vi "LEO PROVA MINCHIATA.vi"() -> ()   [LabVIEW 2014]
uses:
  <vilib>/Platform/TimedLoop/XDataNode/timing_clust.ctl
  <vilib>/Platform/TimedLoop/XDataNode/nitl_modes.ctl
  <vilib>/Platform/TimedLoop/XDataNode/wakeup.ctl
  <vilib>/rvi/Analysis/measure/FFT/simModelSupport/niFPGA FFT Streaming Sim Properties.ctl
  <vilib>/rvi/Analysis/measure/FFT/simModelSupport/niFPGA FFT Sim Stream Group Properties.ctl
  <vilib>/rvi/Analysis/measure/FFT/simModelSupport/niFPGA FFT Sim Types.ctl
  <vilib>/rvi/Analysis/measure/FFT/simModelSupport/niFpgaFFTSimArithmeticProperties.ctl
  <vilib>/rvi/Analysis/measure/FFT/simModelSupport/niFpgaFFTSimDfxp.ctl
  <vilib>/fxp/LVFixedPointQuantizationPolicyTypeDef.ctl
  <vilib>/rvi/Analysis/measure/FFT/XNode/niFpgaFFTButterflyDelays.ctl
  <vilib>/rvi/Emulation/niFpgaSctlEmulationGetInTimedLoop.vi
  <vilib>/rvi/Emulation/niFpgaEmulationReportErrorSimple.vi
  <vilib>/rvi/Emulation/niFpgaGetClockAttributes.vi
  <vilib>/rvi/Emulation/niFpgaCriticalErrorInLSC.vi
  <vilib>/rvi/Emulation/niFpgaEmulationIsFPGAContextNoSignature.vi
  <vilib>/rvi/errors/niFpgaSetErrorForExecOnDevCompSimple.vi
  <vilib>/rvi/eio/common/nirviEmuReportErrorAndStop.vi
  <vilib>/rvi/DataTransferAndStorage/Container/Common/niFpgaContainerGetUniqueNameForEmu.vi
  <vilib>/rvi/FIFO/Fifo_Resource/nirvififoEmulationSetSize.vi
  <vilib>/rvi/FIFO/Fifo_Resource/nirviFifoEmulationQueueMgr.vi
  <instcachedir>/0/nirviFifoEmulationQueueMgr_E5CAEC123FF24DC58D834DCA3CDAA9B5.lvgen/nirviFifoEmulationQueueMgr_E5CAEC123FF24DC58D834DCA3CDAA9B5_012.vi
  <vilib>/rvi/FIFO/Fifo_Resource/nirvififoEmulationCreateLock.vi
  <vilib>/rvi/Emulation/niFpgaProcessEmulError.vi
  <vilib>/rvi/FIFO/Fifo_Resource/nirvififoEmulationObtainLock.vi
  <vilib>/rvi/FIFO/Fifo_Resource/nirvififoEmulationReleaseLock.vi
  <vilib>/rvi/occurrence/nirviWaitOnOccurrenceBase.vi
  <vilib>/rvi/errors/nirviReportUnexpectedCaseInternalError.vi
  <vilib>/rvi/errors/nirviReportUnexpectedCaseInternalError (U32).vi
  <vilib>/rvi/Memory/Memory_Emulation/niFpgaMemoryEmulationCacheClearOnFirstRun.vi
  <vilib>/rvi/Memory/Memory_Emulation/nirvimemoryEmulationManagerCache_MakeExclusive.vi
  <vilib>/rvi/Memory/Memory_Emulation/niFpgaMemoryEmulationValidateCache.vi
  <vilib>/rvi/Memory/Memory_Emulation/nirvimemoryEmulationManagerCache_InsertValue.vi
  <vilib>/Utility/error.llb/Clear Errors.vi
  <vilib>/rvi/Memory/Memory_Emulation/nirvimemoryEmulationManagerCache_ReleaseExclusive.vi
  <vilib>/rvi/Memory/Memory_Emulation/nirvimemoryEmulationManagerCache_GetValue.vi
  <vilib>/rvi/Memory/Memory_Emulation/nirvimemoryEmulationManagerCache_SetValue.vi
  <instcachedir>/0/nirviFifoEmulationQueueMgr_E5CAEC123FF24DC58D834DCA3CDAA9B5.lvgen/nirviFifoEmulationQueueMgr_E5CAEC123FF24DC58D834DCA3CDAA9B5_010.vi
  <vilib>/rvi/FIFO/Fifo_Resource/nirvififoEmulationDetermineInputValidOut.vi
  <vilib>/rvi/Memory/Memory_Emulation/nirvimemoryFastEmulation.vi
  <vilib>/rvi/Memory/Memory_Emulation/nirvimemoryEmulation.vi
  <vilib>/rvi/Analysis/measure/FFT/simModelSupport/niFpgaFFTSimModelStreamingCore.vi
  <vilib>/rvi/interface/RandomDataEmulation/niFpgaRandomDataHandleErrors.vi
  <vilib>/rvi/eio/common/nirviEmuTemplateMethod_errors.vi
  <vilib>/Platform/TimedLoop/XDataNode/XDataNode.xnode
  <vilib>/rvi/DataTransferAndStorage/Container/XNode/niFpgaContainer.xnode
  <vilib>/rvi/FIFO/Fifo_Resource/nirvififoEmulationRead.vi
  <vilib>/rvi/DataTransferAndStorage/Register/Emulation/niFpgaRegisterEmulation.vi
  <vilib>/rvi/FIFO/Fifo_Resource/nirvififoEmulationWrite.vi
  <vilib>/rvi/FIFO/Fifo_Resource/nirvififoEmulationGetNumberOfElementsToWrite.vi
  <vilib>/rvi/Analysis/measure/FFT/XNode/niFpgaFFT.xnode
  <vilib>/rvi/interface/RandomDataEmulation/nirviRandomDataFpgaReadWriteTemplate.vi
  <vilib>/eio/EIOMethodNode/EIOMethodNode.xnode
  <vilib>/Platform/TimedLoop/XDataNode/XDNodeRunTimeDep.lvlib
panel:
  in  "snapshot":bool
  in  "first bin":i32=4
  in  "last bin":i32=251
  in  "lower limit 2":u32=682
  in  "lower limit 1":u32=57
  in  "upper limit 2":u32=1194
  in  "upper limit 1":u32=569
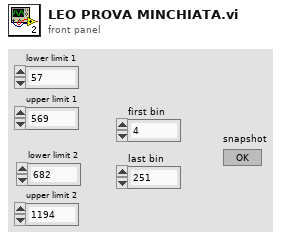
[diagram p1: front panel]
types:
  T1 = typedef "XDNodeRunTimeDep.lvlib/timing_clust.ctl" = cluster{"Expected End [f-1]":u64, "Actual End [f-1]":u64, "Finished Late? [f-1]":bool, "Expected End [i-1]":u64, "Actual End [i-1]":u64, "Finished Late? [i-1]":bool, "Expected Start [i]":u64, "Actual Start [i]":u64, "Expected Start [f]":u64, "Actual Start [f]":u64, "Source Name":string, "Structure Name":string, "Period":i64, "Deadline":i64, "Offset":i64, "Start":i64, "Priority":i32, "Timeout":i32, "Mode":T2, "Wakeup Reason":T3, "Error":errorcluster, "Source Type":string, "Secondary Source Type":string, "Global End Time":u64, "Global Start Time":u64, "Frame Duration":u64, "Iteration Duration":u64, "Assigned CPU":i32, "I/O Scan Engine Mode":u32}
  T2 = typedef "XDNodeRunTimeDep.lvlib/nitl_modes.ctl" = enum32{"No Change", "Process missed periods, maintain original phase", "Discard missed periods, maintain original phase", "Process missed periods, ignore original phase", "Discard missed periods, ignore original phase"}
  T3 = typedef "XDNodeRunTimeDep.lvlib/wakeup.ctl" = enum32{"Normal", "Aborted", "Asynchronous wakeup", "Timing source error", "Timed loop error", "Timeout"}
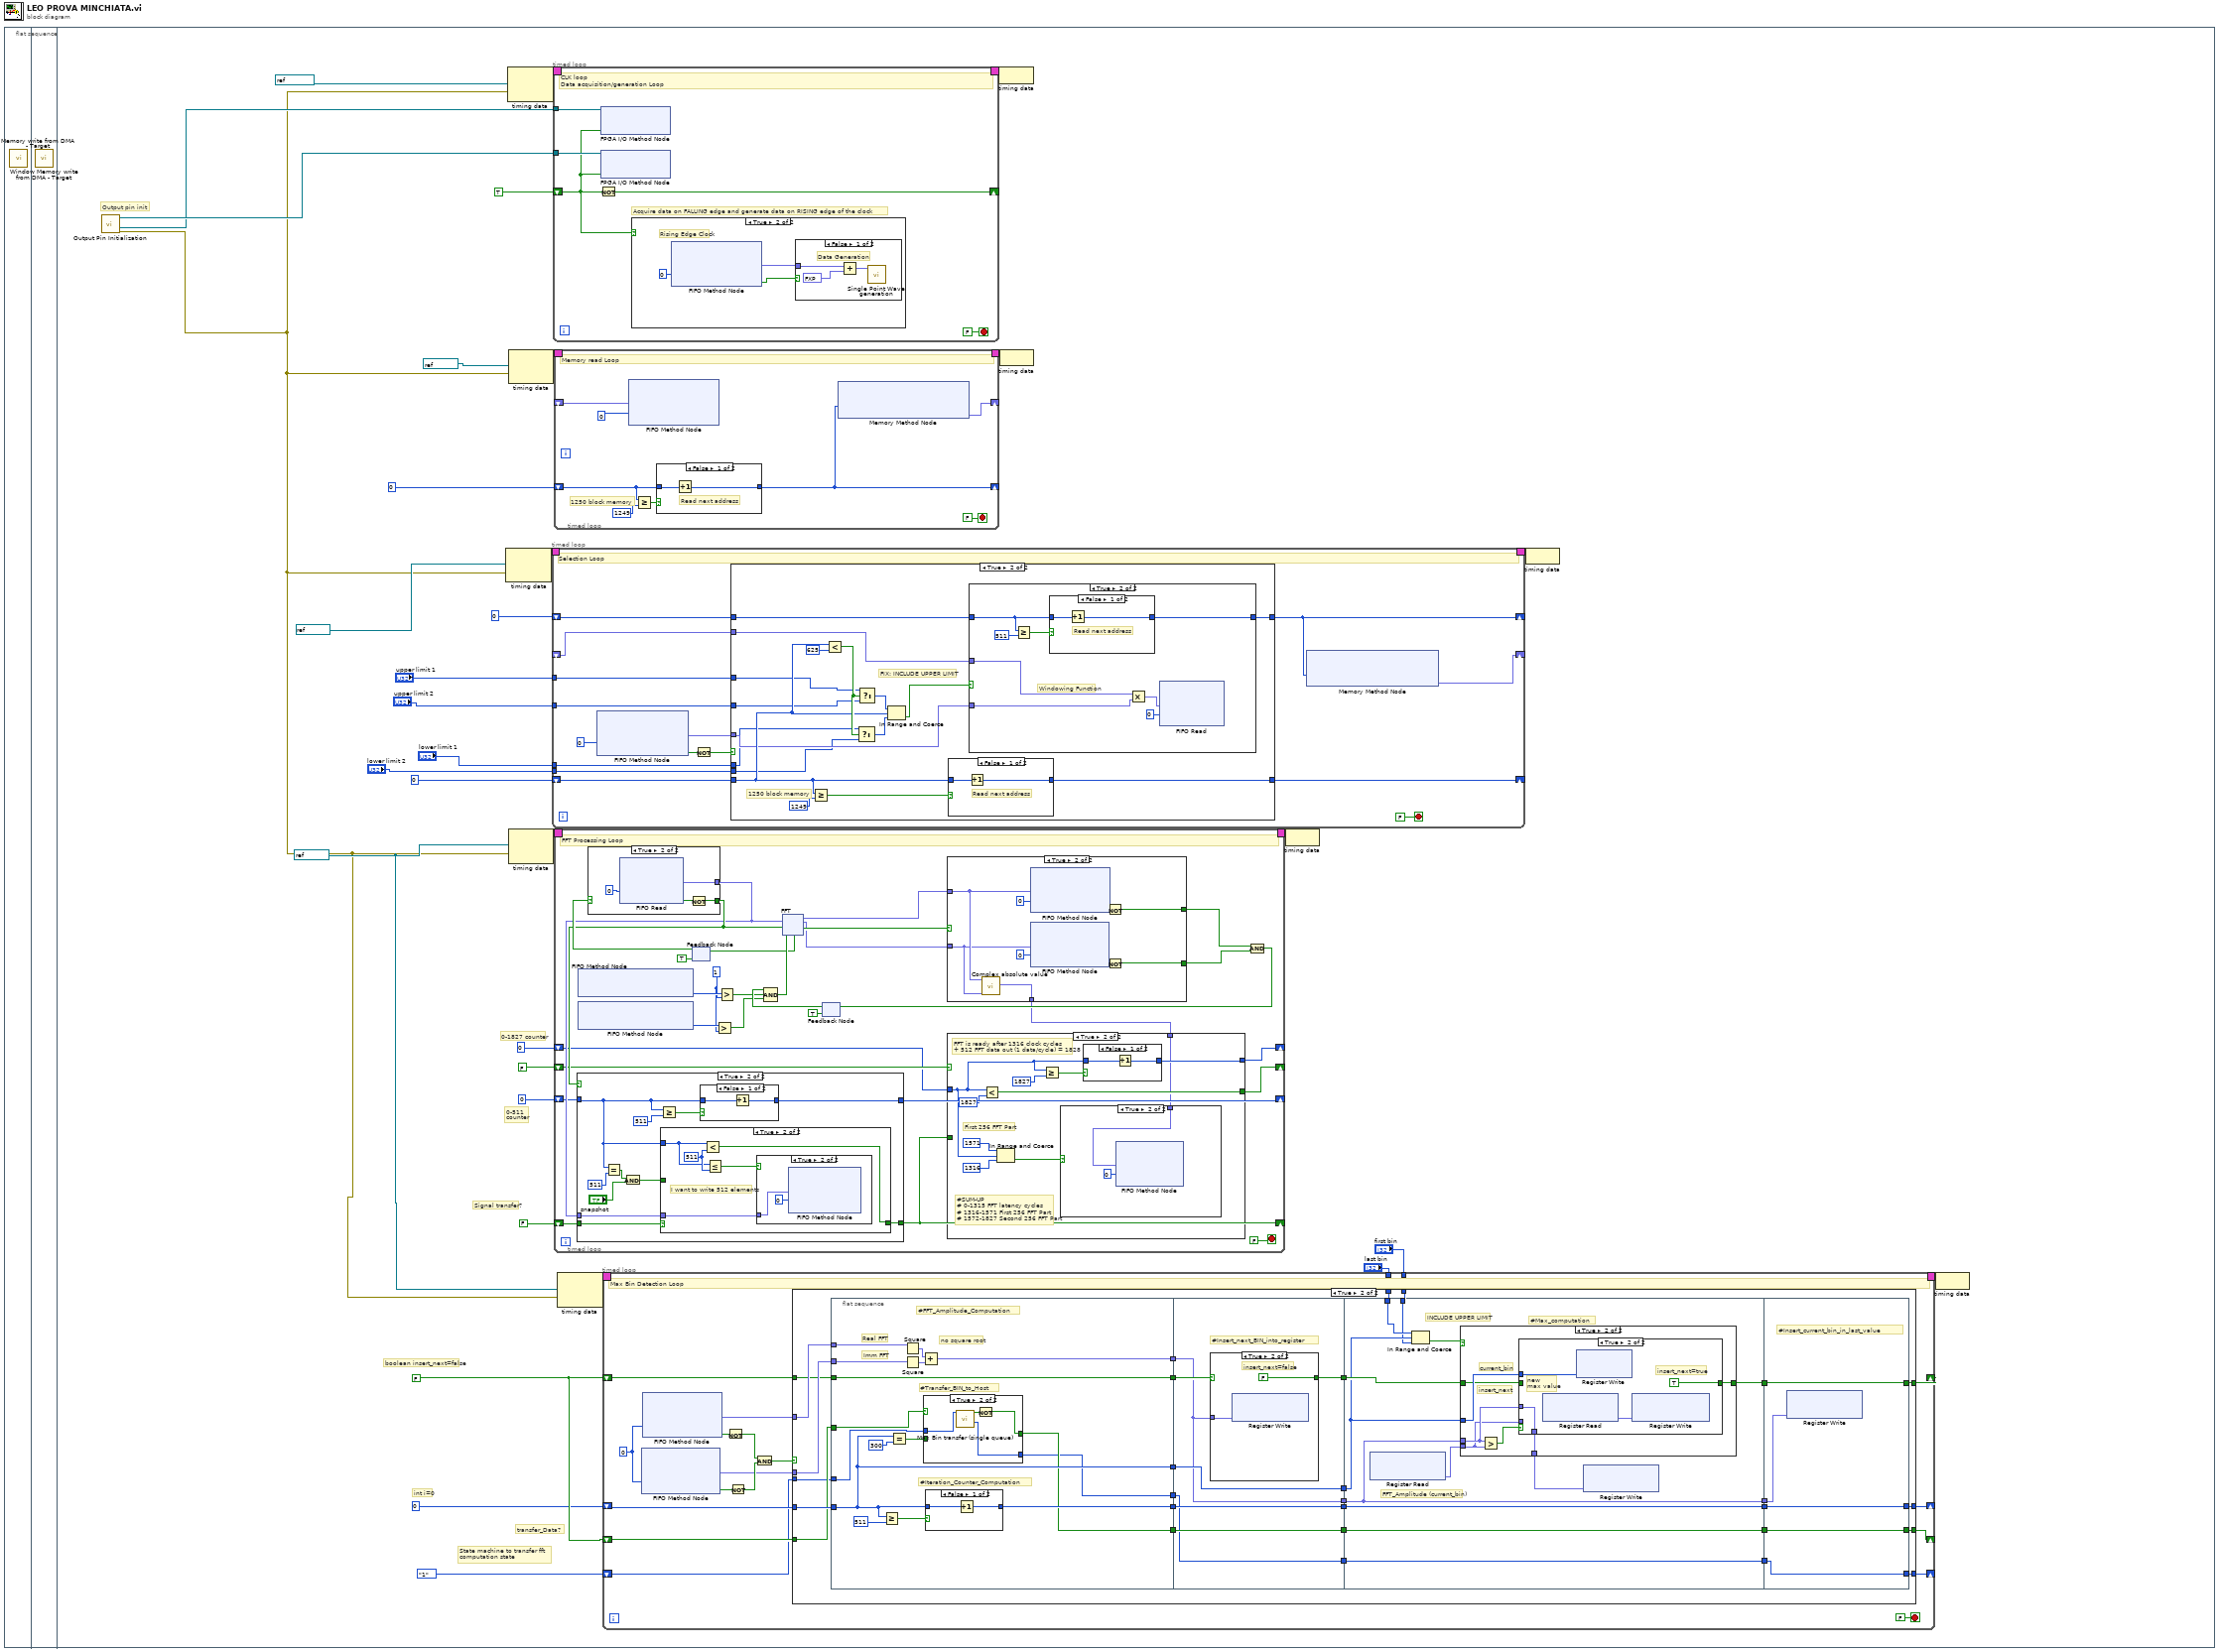
[diagram p0: block diagram]
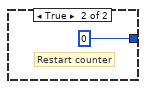
[diagram p4: hidden frame]
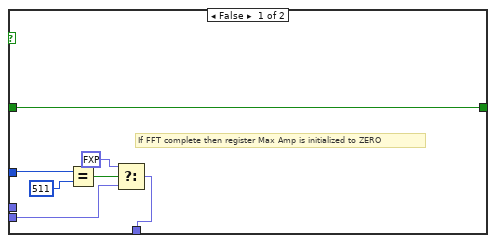
[diagram p6: hidden frame]
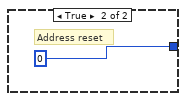
[diagram p10: hidden frame]
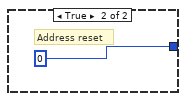
[diagram p11: hidden frame]
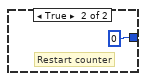
[diagram p14: hidden frame]
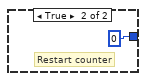
[diagram p18: hidden frame]
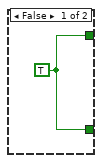
[diagram p19: hidden frame]
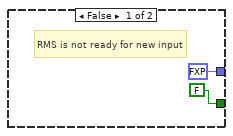
[diagram p20: hidden frame]
diagram:
  n1 = flat-sequence {
    frame #0 {
      n2 = call "Memory write from DMA - Target.vi"() -> ()  [unwired: 12 in]
    }
    frame #1 {
      n3 = call "Window Memory write from DMA - Target.vi"() -> ()  [unwired: 12 in]
    }
    frame #2 {
      w7 = FALSE
      w16 = refnum<k21> "50MHz" ("Source Name")
      # "0-1827 counter"
      # "0-511\ncounter"
      # "Signal transfer?"
      # "State machine to transfer fft\ncomputation state"
      # "transfer_Data?"
      # "int i=0"
      # "boolean insert_next=false"
      # "Output pin init"
      n4 = call "Output Pin Initialization.vi"() -> ("error out"=w15:errorcluster, "I/O Out Clock DAC (pin16)"=w19:refnum<k21>, "I/O Out Clock ADC (pin17)"=w20:refnum<k21>)  [unwired: 8 in]
      n5 = node-c288(refnum<k21> "50MHz" ("Source Name"), w15) -> (w28:T1)
      n6 = node-c288(refnum<k21> "100MHz" ("Source Name"), w15) -> (w34:T1)
      n7 = node-c288(refnum<k21> "50MHz" ("Source Name"), w15) -> (w32:T1)
      n8 = node-c288(w16, w15) -> (w30:T1)
      n9 = timed-loop {
        timing: w28 -> [_]
        timing-out: [_] -> w27
        shift-right: [w179] -> _
        shift-left: u32 0 -> [w178]
        tunnel: "upper limit 1" -> [w173]
        tunnel: "upper limit 2" -> [w172]
        tunnel: "lower limit 1" -> [w171]
        tunnel: "lower limit 2" -> [w170]
        shift-right: [w166] -> _
        shift-left: u32 0 -> [w169]
        shift-right: [w167] -> _
        shift-left: _ -> [w168]
        stop <- FALSE stop-if-true
        # "Selection Loop"
        n10 = xnode ("FIFO Method Node")("Timeout"=0) -> ("Element"=w175:fxp<+/-,12,12>, "Timed Out?"=w176:bool)  [unwired: 1 in, 1 out]
        n11 = Not(x=w176) -> (.not. x?=w177:bool)
        n12 = case shown="True" w177 {
          tunnel: [w182 w197] -> w179
          tunnel: w178 -> [w182 w192]
          tunnel: w175 -> [_ w190]
          tunnel: w173 -> [_ w189]
          tunnel: w172 -> [_ w188]
          tunnel: w171 -> [_ w187]
          tunnel: w170 -> [_ w186]
          tunnel: w169 -> [w181 w183]
          tunnel: [w181 w185] -> w166
          tunnel: w168 -> [_ w184]
          frame False {
          }
          frame True {
            # "FIX: INCLUDE UPPER LIMIT"
            # "1250 block memory"
            n13 = Greater Or Equal?(x=w192, y=u32 1249) -> (x >= y?=w198:bool)
            n14 = Less?(x=w192, y=u32 625) -> (x < y?=w193:bool)
            n15 = Select(t=w187, s=w193, f=w186) -> (s? t:f=w195:u32)
            n16 = Select(t=w189, s=w193, f=w188) -> (s? t:f=w196:u32)
            n17 = In Range and Coerce(upper limit=w196, x=w192, lower limit=w195) -> (In Range?=w191:bool)  [unwired: 1 out]
            n18 = case shown="False" w198 {
              tunnel: w192 -> [w213 _]
              tunnel: [w212 u32 0] -> w197
              frame False {
                # "Read next address"
                n19 = Increment(x=w213) -> (x+1=w212:u32)
              }
              frame True {
                # "Address reset"
              }
            }
            n20 = case shown="True" w191 {
              tunnel: w190 -> [_ w201]
              tunnel: w183 -> [w200 w206]
              tunnel: [w200 w208] -> w185
              tunnel: w184 -> [_ w204]
              frame False {
              }
              frame True {
                # "Windowing Function"
                n21 = Greater Or Equal?(x=w206, y=u32 511) -> (x >= y?=w207:bool)
                n22 = case shown="False" w207 {
                  tunnel: w206 -> [w210 _]
                  tunnel: [w209 u32 0] -> w208
                  frame False {
                    # "Read next address"
                    n23 = Increment(x=w210) -> (x+1=w209:u32)
                  }
                  frame True {
                    # "Address reset"
                  }
                }
                n24 = Multiply(x=w204, y=w201) -> (x*y=w202:fxp<+/-,12,12>)
                n25 = xnode ("FIFO Read")("Element"=w202, "Timeout"=0) -> ()  [unwired: 1 in, 2 out]
              }
            }
          }
        }
        n26 = xnode ("Memory Method Node")("Address"=w166) -> ("Data"=w167:fxp<+,8,1>)  [unwired: 1 in, 1 out]
      }
      n27 = timed-loop {
        timing: w34 -> [_]
        timing-out: [_] -> w33
        shift-right: [w361] -> _
        shift-left: TRUE -> [w359]
        tunnel: w19 -> [w363]
        tunnel: w20 -> [w360]
        stop <- FALSE stop-if-true
        # "Acquire data on FALLING edge and generate data on RISING edge of the clock"
        # "CLK loop\nData acquisition/generation Loop"
        n28 = Not(x=w359) -> (.not. x?=w361:bool)
        n29 = xnode "FPGA I/O Method Node"("FPGA I/O In"=w363, "Data"=w359) -> ()  [unwired: 1 out]
        n30 = xnode "FPGA I/O Method Node"("FPGA I/O In"=w360, "Data"=w359) -> ()  [unwired: 1 out]
        n31 = case shown="True" w359 {
          frame False {
            # "Falling Edge Clock"
            n32 = call "Single Acquisition.vi"() -> ("Out"=w365:fxp<+/-,12,12>)  [unwired: 10 in, 1 out]
            n33 = xnode ("FIFO Method Node")("Element"=w365, "Timeout"=0) -> ()  [unwired: 1 in, 2 out]
          }
          frame True {
            # "Rising Edge Clock"
            n34 = xnode ("FIFO Method Node")("Timeout"=0) -> ("Element"=w366:fxp<+/-,12,12>, "Timed Out?"=w367:bool)  [unwired: 1 in, 1 out]
            n35 = case shown="False" w367 {
              tunnel: w366 -> [w371 _]
              frame False {
                # "Data Generation"
                n36 = Add(x=w371, y=fxp<+,12,12> 2048.0) -> (x+y=w369:fxp<+/-,14,14>)
                n37 = call "Single Point Wave generation.vi"("Data To Write"=w369) -> ()  [unwired: 10 in, 1 out]
              }
              frame True {
                # "FPGA memory slow"
              }
            }
          }
        }
      }
      n38 = timed-loop {
        timing: w32 -> [_]
        timing-out: [_] -> w31
        shift-right: [w341] -> _
        shift-left: u32 0 -> [w345]
        shift-right: [w343] -> _
        shift-left: _ -> [w342]
        stop <- FALSE stop-if-true
        # "1250 block memory"
        # "Memory read Loop"
        n39 = xnode ("FIFO Method Node")("Element"=w342, "Timeout"=0) -> ()  [unwired: 1 in, 2 out]
        n40 = Greater Or Equal?(x=w345, y=u32 1249) -> (x >= y?=w347:bool)
        n41 = case shown="False" w347 {
          tunnel: w345 -> [w350 _]
          tunnel: [w349 u32 0] -> w341
          frame False {
            # "Read next address"
            n42 = Increment(x=w350) -> (x+1=w349:u32)
          }
          frame True {
            # "Address reset"
          }
        }
        n43 = xnode ("Memory Method Node")("Address"=w341) -> ("Data"=w343:fxp<+/-,12,12>)  [unwired: 1 in, 1 out]
      }
      n44 = timed-loop {
        timing: w30 -> [_]
        timing-out: [_] -> w29
        shift-right: [w227] -> _
        shift-left: FALSE -> [w230]
        shift-right: [w231] -> _
        shift-left: i16 0 -> [w228]
        shift-right: [w226] -> _
        shift-left: FALSE -> [w225]
        shift-right: [w223] -> _
        shift-left: i16 0 -> [w224]
        stop <- FALSE stop-if-true
        w235 = u32 1 ("y")
        # "FFT Processing Loop"
        n45 = xnode ("FIFO Method Node")() -> ("Number of Elements to Write"=w237:u32)  [unwired: 1 in, 1 out]
        n46 = xnode ("FIFO Method Node")() -> ("Number of Elements to Write"=w236:u32)  [unwired: 1 in, 1 out]
        n47 = feedback #1(TRUE ("ready for input")) -> (w250:bool)
        n48 = case shown="True" w250 {
          tunnel: [FALSE w333] -> w232
          tunnel: [fxp<+/-,12,12> 0.0 ("Element") w330] -> w229
          frame False {
            # "RMS is not ready for new input"
          }
          frame True {
            n49 = xnode ("FIFO Read")("Timeout"=0) -> ("Element"=w330:fxp<+/-,12,12>, "Timed Out?"=w332:bool)  [unwired: 1 in, 1 out]
            n50 = Not(x=w332) -> (.not. x?=w333:bool)
          }
        }
        n51 = case shown="True" w232 {
          tunnel: w228 -> [w269 w273]
          tunnel: [w269 w278] -> w231
          tunnel: w230 -> [w268 w271]
          tunnel: [w268 w272] -> w227
          tunnel: w229 -> [_ w270]
          frame False {
          }
          frame True {
            n52 = Equal?(x=w273, y=i16 511) -> (x = y?=w277:bool)
            n53 = And(x=w277, y="snapshot") -> (x .and. y?=w274:bool)
            n54 = Greater Or Equal?(x=w273, y=i16 511) -> (x >= y?=w279:bool)
            n55 = case shown="True" w271 {
              tunnel: w274 -> [w281 _]
              tunnel: w273 -> [_ w282]
              tunnel: [w281 w286] -> w272
              tunnel: w270 -> [_ w284]
              frame False {
              }
              frame True {
                w283 = i16 511 ("y")
                # "I want to write 512 elements"
                n56 = Less?(x=w282, y=w283) -> (x < y?=w286:bool)
                n57 = Less Or Equal?(x=w282, y=w283) -> (x <= y?=w285:bool)
                n58 = case shown="True" w285 {
                  tunnel: w284 -> [_ w287]
                  frame False {
                  }
                  frame True {
                    n59 = xnode ("FIFO Method Node")("Element"=w287, "Timeout"=0) -> ()  [unwired: 1 in, 2 out]
                  }
                }
              }
            }
            n60 = case shown="False" w279 {
              tunnel: w273 -> [w290 _]
              tunnel: [w289 i16 0] -> w278
              frame False {
                n61 = Increment(x=w290) -> (x+1=w289:i16)
              }
              frame True {
                # "Restart counter"
              }
            }
          }
        }
        n62 = Greater?(x=w236, y=w235) -> (0:w233:bool)
        n63 = Greater?(x=w237, y=w235) -> (0:w234:bool)
        n64 = feedback #2(TRUE) -> (w246:bool)
        n65 = Compound Arithmetic op=AND(w246, w234, w233) -> (w245:bool)
        n66 = xnode "FFT"("real data in"=w229, "input valid"=w232, "ready for output"=w245) -> ("ready for input"=w244:bool, "real data out"=w242:fxp<+/-,22,22>, "imaginary data out"=w241:fxp<+/-,22,22>, "output valid"=w243:bool)  [unwired: 2 in, 1 out]
        n67 = feedback-in #1(w244) -> ()
        n68 = case shown="True" w243 {
          tunnel: w242 -> [_ w321]
          tunnel: w241 -> [_ w320]
          tunnel: [w318 w327] -> w240
          tunnel: [w318 w326] -> w239
          tunnel: [_ w319] -> w222
          frame False {
            w318 = TRUE
          }
          frame True {
            n69 = call "Complex absolute value.vi"("Im"=w320, "Re"=w321) -> ("Square Absolute Value"=w319:fxp<+,44,44>)  [unwired: 9 in]
            n70 = xnode ("FIFO Method Node")("Element"=w321, "Timeout"=0) -> ("Timed Out?"=w322:bool)  [unwired: 1 in, 1 out]
            n71 = xnode ("FIFO Method Node")("Element"=w320, "Timeout"=0) -> ("Timed Out?"=w323:bool)  [unwired: 1 in, 1 out]
            n72 = Not(x=w322) -> (.not. x?=w327:bool)
            n73 = Not(x=w323) -> (.not. x?=w326:bool)
          }
        }
        n74 = case shown="True" w225 {
          tunnel: w227 -> [w252 _]
          tunnel: [w252 w262] -> w226
          tunnel: w224 -> [w251 w255]
          tunnel: [w251 w258] -> w223
          tunnel: w222 -> [_ w253]
          frame False {
          }
          frame True {
            # "First 256 FFT Part"
            # "#SUM-UP\n# 0-1315 FFT latency cycles\n# 1316-1571 First 256 FFT Part\n# 1572-1827 Second 256 FFT Part"
            # "FFT is ready after 1316 clock cycles\n+ 512 FFT data out (1 data/cycle) = 1828"
            n75 = Less?(x=w255, y=i16 1827) -> (x < y?=w262:bool)
            n76 = In Range and Coerce(upper limit=i16 1571, x=w255, lower limit=i16 1316 ("y")) -> (In Range?=w254:bool)  [unwired: 1 out]
            n77 = Greater Or Equal?(x=w255, y=i16 1827) -> (x >= y?=w259:bool)
            n78 = case shown="True" w254 {
              tunnel: w253 -> [_ w264]
              frame False {
              }
              frame True {
                n79 = xnode ("FIFO Method Node")("Element"=w264, "Timeout"=0) -> ()  [unwired: 1 in, 2 out]
              }
            }
            n80 = case shown="False" w259 {
              tunnel: w255 -> [w266 _]
              tunnel: [w265 i16 0] -> w258
              frame False {
                n81 = Increment(x=w266) -> (x+1=w265:i16)
              }
              frame True {
                # "Restart counter"
              }
            }
          }
        }
        n82 = Compound Arithmetic op=AND(w240, w239) -> (w238:bool)
        n83 = feedback-in #2(w238) -> ()
      }
      n84 = node-c288(w16, w15) -> (w26:T1)
      n85 = timed-loop {
        shift-right: [w45] -> _
        shift-left: 0 ("Timeout") -> [w46]
        shift-right: [w43] -> _
        shift-left: w7 -> [w44]
        timing: w26 -> [_]
        timing-out: [_] -> w25
        tunnel: "last bin" -> [w41]
        tunnel: "first bin" -> [w40]
        shift-right: [w37] -> _
        shift-left: w7 -> [w38]
        shift-right: [w35] -> _
        shift-left: enum16{"1", "2", "3", "4"}."1" ("Enum") -> [w36]
        stop <- FALSE stop-if-true
        w39 = 0 ("Timeout")
        # "Max Bin Detection Loop"
        n86 = xnode ("FIFO Method Node")("Timeout"=w39) -> ("Element"=w47:fxp<+/-,22,22>, "Timed Out?"=w52:bool)  [unwired: 1 in, 1 out]
        n87 = xnode ("FIFO Method Node")("Timeout"=w39) -> ("Element"=w48:fxp<+/-,22,22>, "Timed Out?"=w53:bool)  [unwired: 1 in, 1 out]
        n88 = Not(x=w53) -> (.not. x?=w51:bool)
        n89 = Not(x=w52) -> (.not. x?=w50:bool)
        n90 = And(x=w51, y=w50) -> (x .and. y?=w49:bool)
        n91 = case shown="True" w49 {
          tunnel: w48 -> [_ w86]
          tunnel: w47 -> [_ w85]
          tunnel: w46 -> [w57 w83]
          tunnel: [w57 w70] -> w45
          tunnel: w44 -> [w56 w77]
          tunnel: [w56 w72] -> w43
          tunnel: w41 -> [_ w69]
          tunnel: w40 -> [_ w68]
          tunnel: w38 -> [w55 w67]
          tunnel: [w55 w66] -> w37
          tunnel: w36 -> [w54 w62]
          tunnel: [w54 w58] -> w35
          frame False {
            # "Data are NOT ready in Target Real FFT and Target Imm FFT FIFOs"
          }
          frame True {
            n92 = flat-sequence {
              tunnel: w86 -> [w99]
              tunnel: w85 -> [w100]
              tunnel: [w93] -> w84
              tunnel: w83 -> [w92]
              tunnel: [w98] -> w82
              tunnel: [w92] -> w79
              tunnel: [w95] -> w78
              tunnel: w77 -> [w95]
              tunnel: w67 -> [w91]
              tunnel: [w89] -> w65
              tunnel: w62 -> [w88]
              tunnel: [w87] -> w59
              tunnel: w84 -> [w115]
              tunnel: w82 -> [w118]
              tunnel: [w118] -> w81
              tunnel: w79 -> [w116]
              tunnel: w78 -> [w117]
              tunnel: [w116] -> w76
              tunnel: [w115] -> w75
              tunnel: [w114] -> w74
              tunnel: w65 -> [w113]
              tunnel: [w113] -> w64
              tunnel: [w112] -> w60
              tunnel: w59 -> [w112]
              tunnel: w81 -> [w133]
              tunnel: [w133] -> w80
              tunnel: w76 -> [w128]
              tunnel: w75 -> [w130]
              tunnel: w74 -> [w131]
              tunnel: [w130] -> w73
              tunnel: [w129] -> w71
              tunnel: w69 -> [w125]
              tunnel: w68 -> [w124]
              tunnel: w64 -> [w123]
              tunnel: [w123] -> w63
              tunnel: [w122] -> w61
              tunnel: w60 -> [w122]
              tunnel: w80 -> [w156]
              tunnel: w73 -> [w158]
              tunnel: w71 -> [w157]
              tunnel: [w157] -> w72
              tunnel: [w156] -> w70
              tunnel: [w155] -> w66
              tunnel: w63 -> [w155]
              tunnel: w61 -> [w154]
              tunnel: [w154] -> w58
              frame #0 {
                # "no square root"
                # "#Transfer_BIN_to_Host"
                # "#Iteration_Counter_Computation"
                # "#FFT_Amplitude_Computation"
                # "Imm FFT"
                # "Real FFT"
                n93 = Greater Or Equal?(x=w92, y=511) -> (x >= y?=w96:bool)
                n94 = Equal?(x=w92, y=300) -> (x = y?=w90:bool)
                n95 = Square(x=w99) -> (x^2=w102:fxp<+,43,43>)
                n96 = Square(x=w100) -> (x^2=w101:fxp<+,43,43>)
                n97 = Add(x=w102, y=w101) -> (x+y=w93:fxp<+,44,44>)
                n98 = case shown="True" w91 {
                  tunnel: w90 -> [w104 _]
                  tunnel: [w104 w107] -> w89
                  tunnel: w88 -> [w103 w106]
                  tunnel: [w103 w105] -> w87
                  frame False {
                    # "FFT Comp is NOT finished"
                  }
                  frame True {
                    n99 = call "Max Bin transfer (single queue).vi"("Enum"=w106) -> ("Next state"=w105:enum16{"1", "2", "3", "4"}, "END?"=w108:bool)  [unwired: 9 in]
                    n100 = Not(x=w108) -> (.not. x?=w107:bool)
                  }
                }
                n101 = case shown="False" w96 {
                  tunnel: w92 -> [w109 _]
                  tunnel: [w110 0 ("Timeout")] -> w98
                  frame False {
                    n102 = Increment(x=w109) -> (x+1=w110:i32)
                  }
                  frame True {
                    # "Restart counter"
                  }
                }
              }
              frame #1 {
                # "#Insert_next_BIN_into_register"
                n103 = case shown="True" w117 {
                  selector: w117 -> [w119 _]
                  tunnel: [w119 FALSE] -> w114
                  tunnel: w115 -> [_ w120]
                  frame False {
                  }
                  frame True {
                    # "insert_next=false"
                    n104 = xnode ("Register Write")("Data"=w120) -> ()  [unwired: 1 in, 1 out]
                  }
                }
              }
              frame #2 {
                # "INCLUDE UPPER LIMIT"
                # "FFT_Amplitude (current_bin)"
                # "#Max_computation"
                n105 = xnode ("Register Read")() -> ("Data"=w127:fxp<+,44,44>)  [unwired: 1 in, 1 out]
                n106 = In Range and Coerce(upper limit=w125, x=w128, lower limit=w124) -> (In Range?=w132:bool)  [unwired: 1 out]
                n107 = case shown="True" w132 {
                  tunnel: w130 -> [_ w146]
                  tunnel: w128 -> [w138 w145]
                  tunnel: w131 -> [w140 w144]
                  tunnel: [w140 w143] -> w129
                  tunnel: w127 -> [w136 w141]
                  tunnel: [w134 w142] -> w126
                  frame False {
                    # "If FFT complete then register Max Amp is initialized to ZERO"
                    n108 = Equal?(x=w138, y=511) -> (x = y?=w139:bool)
                    n109 = Select(t=fxp<+,44,44> 0.0, s=w139, f=w136) -> (s? t:f=w134:fxp<+,44,44>)
                  }
                  frame True {
                    # "insert_next"
                    # "current_bin"
                    n110 = Greater?(x=w146, y=w141) -> (0:w147:bool)
                    n111 = case shown="True" w147 {
                      tunnel: w146 -> [_ w150]
                      tunnel: w145 -> [_ w153]
                      tunnel: w144 -> [w149 _]
                      tunnel: [w149 TRUE] -> w143
                      tunnel: [w148 w150] -> w142
                      tunnel: w141 -> [w148 _]
                      frame False {
                        # "Old value is re-written"
                      }
                      frame True {
                        # "new\nmax value"
                        # "insert_next=true"
                        n112 = xnode ("Register Read")() -> ("Data"=w151:fxp<+,44,44>)  [unwired: 1 in, 1 out]
                        n113 = xnode ("Register Write")("Data"=w153) -> ()  [unwired: 1 in, 1 out]
                        n114 = xnode ("Register Write")("Data"=w151) -> ()  [unwired: 1 in, 1 out]
                      }
                    }
                  }
                }
                n115 = xnode ("Register Write")("Data"=w126) -> ()  [unwired: 1 in, 1 out]
              }
              frame #3 {
                # "#Insert_current_bin_in_last_value"
                n116 = xnode ("Register Write")("Data"=w158) -> ()  [unwired: 1 in, 1 out]
              }
            }
          }
        }
      }
      n117 = node-c288(w33) -> ()
      n118 = node-c288(w31) -> ()
      n119 = node-c288(w29) -> ()
      n120 = node-c288(w27) -> ()
      n121 = node-c288(w25) -> ()
    }
  }
